vi "Disconnect.vi"(8 "error in":errorcluster, 11 "PowerSupply in":refnum<class "PowerSupply.lvclass">) -> (0 "error out":errorcluster, 3 "PowerSupply out":refnum<class "PowerSupply.lvclass">)   [LabVIEW 2019, in "PowerSupply.lvlib" / "PowerSupply.lvclass"]
doc: "This disconnect routine is a must override from the Instrument Class\nChildren Classes are responsible for handling the override, but the parent class is an intermediary and must contain the override functions to maintain the rules for the method."
uses:
  Library/PowerSupply.lvclass
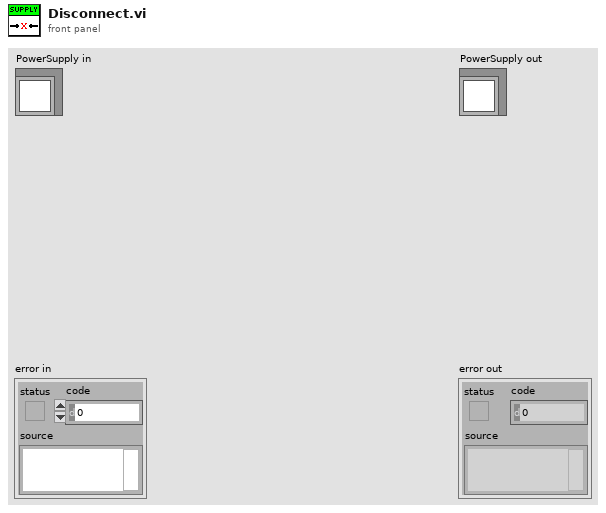
[diagram p1: front panel]
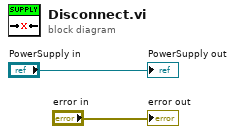
[diagram p0: block diagram]
diagram:
  "error out" <- "error in"
  "PowerSupply out" <- "PowerSupply in"
